vi "Configure State Trigger.vi"(0 "VISA resource name":refnum<visa-resource-name>, 1 "Trigger Slope (0: Rising)":u16(ring) items=["Rising", "Falling"], 2 "Trigger Source (0: Channel 1)":u16(ring) items=["Channel 1", "Channel 2", "Channel 3", "Channel 4", "External", "Line", "Ext", "Ext10"], 3 "Trigger Source After Qualifier (1: Channel 2)":u16(ring)=1 items=["Channel 1", "Channel 2", "Channel 3", "Channel 4", "External", "Line", "Ext", "Ext10"], 5 "Trigger Level (0.0 V)":dbl, 7 "Trigger Level 2 (0.0 V)":dbl, 9 "Holdoff Type(0: TI)":u16(ring) items=["TI", "TL", "Events", "None"], 11 "error in (no error)":errorcluster, 12 "Holdoff Value by Time (10 ns)":dbl=1e-08, 14 "Holdoff Value by Events (1)":i32=1) -> (4 "VISA resource name out":refnum<visa-resource-name>, 15 "error out":errorcluster)   [LabVIEW 2013, in "LeCroy Wave Series.lvlib"]
doc: "Configures state trigger settings. The State trigger is a level-qualified SMART Trigger which requires that the qualifying signal remain above or below a specified voltage level for a trigger to occur. For Sate trigger, you specify the time or number of events after the signal has gone above or below the voltage level when you want the trigger to occur.\n\nNote: \"External\" is included for the purpose of backwards compatibility. Use EXT or EXT10 for best results."
uses:
  LeCroy Wave Series.lvlib
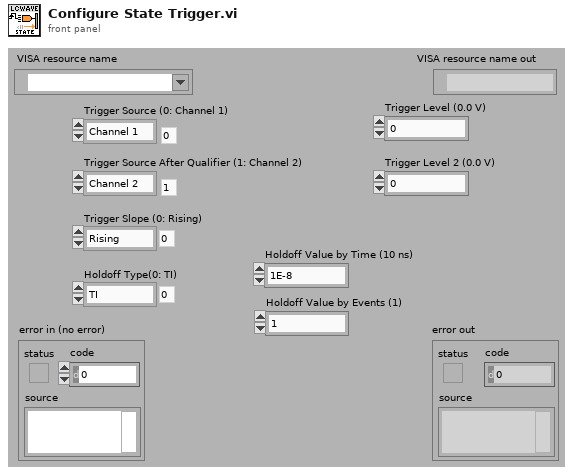
[diagram p1: front panel]
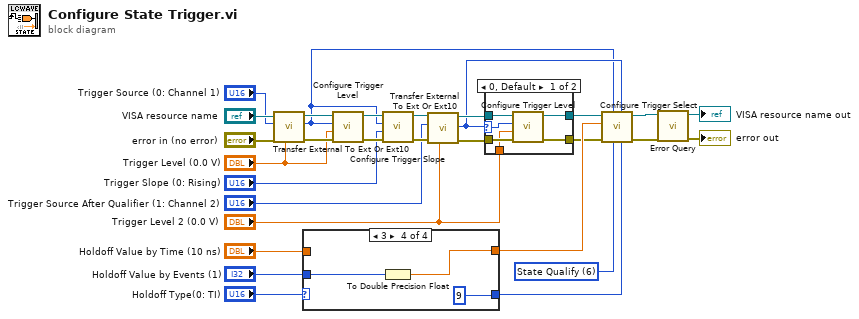
[diagram p0: block diagram]
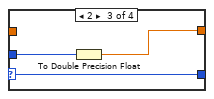
[diagram p5: hidden frame]
diagram:
  w3 = u16 6 items=["Edge", "Dropout", "Glitch", "Interval", "Std", "Sng", "State Qualify", "Edge Qualify"] ("Trigger type")
  n1 = call "Transfer External To Ext Or Ext10.vi"("Trigger Level"="Trigger Level (0.0 V)", "error in (no error)"="error in (no error)", "Trigger Source With External"="Trigger Source (0: Channel 1)", "VISA resource name"="VISA resource name") -> ("error out"=w14:errorcluster, "Trigger Source With Ext/Ext10"=w1:u16, "VISA resource name out"=w15:refnum<visa-resource-name>)  [unwired: 5 in]
  n2 = case shown="3" "Holdoff Type(0: TI)" {
    selector: "Holdoff Type(0: TI)" -> [w30 w32 w36 _]
    tunnel: "Holdoff Value by Events (1)" -> [_ _ w35 w38]
    tunnel: [w31 w33 w34 w37] -> w27
    tunnel: "Holdoff Value by Time (10 ns)" -> [w31 w33 _ _]
    tunnel: [w30 w32 w36 9] -> w25
    frame 0, Default {
    }
    frame 1 {
    }
    frame 2 {
      n3 = To Double Precision Float(number=w35) -> (double precision float=w34:dbl)
    }
    frame 3 {
      n4 = To Double Precision Float(number=w38) -> (double precision float=w37:dbl)
    }
  }
  n5 = call "Configure Trigger Level.vi"("error in (no error)"=w14, "Trigger Level 1 (0.0 V)"="Trigger Level (0.0 V)", "Channel (0: Channel 1)"=w1, "VISA resource name"=w15) -> ("error out"=w19:errorcluster, "VISA resource name out"=w20:refnum<visa-resource-name>)  [unwired: 6 in]
  n6 = call "Configure Trigger Slope.vi"("error in (no error)"=w19, "Trigger Slope (0: Rising)"="Trigger Slope (0: Rising)", "Channel (0: Channel 1)"=w1, "VISA resource name"=w20) -> ("error out"=w8:errorcluster, "VISA resource name out"=w9:refnum<visa-resource-name>)  [unwired: 6 in]
  n7 = call "Transfer External To Ext Or Ext10.vi"("Trigger Level"="Trigger Level 2 (0.0 V)", "error in (no error)"=w8, "Trigger Source With External"="Trigger Source After Qualifier (1: Channel 2)", "VISA resource name"=w9) -> ("error out"=w6:errorcluster, "Trigger Source With Ext/Ext10"=w2:u16, "VISA resource name out"=w7:refnum<visa-resource-name>)  [unwired: 5 in]
  n8 = case shown="0, Default" w2 {
    selector: w2 -> [w40 _]
    tunnel: w7 -> [w45 w47]
    tunnel: w6 -> [w44 w46]
    tunnel: [w43 w47] -> w18
    tunnel: [w42 w46] -> w17
    tunnel: "Trigger Level 2 (0.0 V)" -> [w41 _]
    frame 0, Default {
      n9 = call "Configure Trigger Level.vi"("error in (no error)"=w44, "Trigger Level 1 (0.0 V)"=w41, "Channel (0: Channel 1)"=w40, "VISA resource name"=w45) -> ("error out"=w42:errorcluster, "VISA resource name out"=w43:refnum<visa-resource-name>)  [unwired: 6 in]
    }
    frame 6 {
    }
  }
  n10 = call "Configure Trigger Select.vi"("Hold Type (0: TI)"=w25, "QL (1: Channel 2)"=w2, "Trigger type"=w3, "Trigger Source (0: Channel 1)"=w1, "error in (no error)"=w17, "Hold Value 1 (4 ns)"=w27, "VISA resource name"=w18) -> ("error out"=w21:errorcluster, "VISA resource name out"=w22:refnum<visa-resource-name>)  [unwired: 3 in]
  n11 = call "Error Query.vi"("error in (no error)"=w21, "VISA resource name"=w22) -> ("error out"=→"error out":errorcluster, "VISA resource name out"=→"VISA resource name out":refnum<visa-resource-name>)  [unwired: 6 in, 2 out]
